vi "zgerc - General Matrix Rank-1 Update with Conjugation (CDB).vi"(6 "alpha":cdb=1.0+0.0i, 9 "A":T1, 10 "y":cdb[](array[numeric]), 11 "x":cdb[](array[numeric])) -> (0 "error":i32, 3 "zgerc":T1)   [LabVIEW 2014, in "NI_AALBLAS.lvlib"]
doc: "Calculates the rank-1 conjugated update of a general matrix."
uses:
  NI_AALBLAS.lvlib
  ComplexMatrix.ctl
  Fucntion.ctl
  Order.ctl
  BLAS2 Utility(CDB).vi
  NI_Matrix.lvlib
panel:
  # "zgerc=alpha*x*conjg(y')+A"
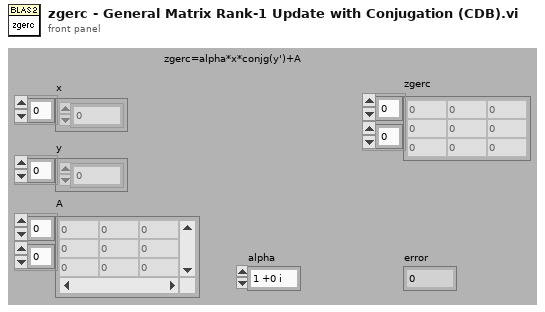
[diagram p1: front panel]
types:
  T1 = typedef "NI_Matrix.lvlib/ComplexMatrix.ctl" = cdb[][]
  T2 = typedef "NI_AALBLAS.lvlib/Order.ctl" = i32
  T3 = typedef "NI_AALBLAS.lvlib/fucntion.ctl" = u16
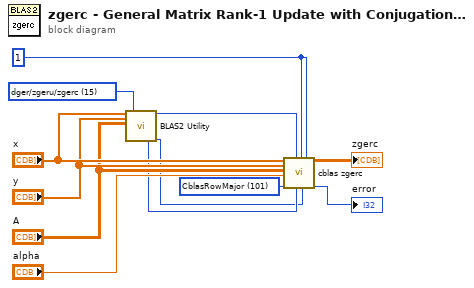
[diagram p0: block diagram]
diagram:
  w3 = 1
  w5 = T2 101 items=["CblasRowMajor"=101, "CblasColMajor"=102] ("order")
  w6 = T3 15 items=["ddot/zdotu/zdotc", "daxpy/zaxpy", "dnrm2/dznrm2", "dasum/dzasum", "dcopy/zcopy", "dswap/zswap", "drotm", "drot/zdrot", "idamax/izamax", "idamin/izamin", "dgemv/zgemv", "dsymv/zhemv", "dtrmv/ztrmv", "dsyr/zher", "dsyr2/zher2", "dger/zgeru/zgerc", "dtrsv/ztrsv", "dgemm/zgemm", "dsymm/zsymm/zhemm", "dtrmm/ztrmm", "dsyrk/zsyrk/zherk", "dsyr2k/zsyr2k/zher2k", "dtrsm/ztrsm"] ("function")
  n1 = call-poly "BLAS2 Utility.vi"("x"="x", "y"="y", "A"="A", "function"=w6) -> ("m"=w2:i32, "lda"=w4:i32, "n"=w1:i32)  [unwired: 1 in, 12 out]
  n2 = call "cblas zgerc.vi"("x"="x", "y"="y", "A"="A", "alpha"="alpha", "order"=w5, "lda"=w4, "m"=w2, "incx"=w3, "n"=w1, "incy"=w3) -> ("zgerc"=→"zgerc":T1, "error"=→"error":i32)  [unwired: 8 out]
